vi "uService GUI.vi"(8 "error in (no error)":errorcluster, 11 "uService Template in":refnum<class "Common GUI v3.lvclass">) -> (3 "uService Template out":refnum<class "Common GUI v3.lvclass">)   [LabVIEW 2026, in "TALOS.lvlib" / "Common GUI v3.lvlib" / "Common GUI v3.lvclass"]
uses:
  Common GUI v3.lvclass
  C:/LabVIEW Code/TALOS/talos/Father of all uServices/Father of all uServices/Father of all uServices.lvclass
  Ancestor/Ancestor/Ancestor.lvclass/Ancestor.ctl
  Support VIs/Substitute Error.vi
  Support VIs/Generate Error.vi
  FGV/Error Memory/Get Error Description.vi
  Support VIs/Get PC name.vi
  Ancestor/Ancestor/Read ID.vi
  Support VIs/Get Class Name.vi
  FGV/Error Memory/Error Memory Core.vi
  <vilib>/AdvancedString/Delimited String to 1D String Array.vi
  <vilib>/AdvancedString/Delimited String to 1D String Array (string).vi
  Support VIs/Circus Root Path.vi
  FGV/Error Memory/Error Crt Lvl checker.vi
  FGV/Error Memory/Error Memory Core.vi/40c8088d-b597-4017-91af-faa98e00292e.vi
  FGV/Error Memory/Error Memory Core.vi/d4a3ab98-063c-4e44-b43d-fbdcfe6c2be2.vi
  Father of all uServices/Father of all uServices/Father of all uServices.lvclass
  C:/LabVIEW Code/TALOS/builds/Actor Framework PPL/Actor Framework.lvlibp/1abvi3w/vi.lib/ActorFramework/Actor/Actor.lvclass
  builds/Actor Framework PPL/Actor Framework.lvlibp/1abvi3w/vi.lib/ActorFramework/Actor/Read Self Enqueuer.vi
  builds/Actor Framework PPL/Actor Framework.lvlibp/1abvi3w/vi.lib/ActorFramework/Stop Msg/Send Normal Stop.vi
  Support VIs/Global Memory.vi
  <vilib>/Utility/LVClass/Get LV Class Name.vi
  Support VIs/Is in Packed Library.vi
  Support VIs/TALOS Root path.vi
  Support VIs/Read CSV worksheet.vi
  Support VIs/Global Constants.vi
  <vilib>/Utility/error.llb/General Error Handler.vi
  Support VIs/Error Log.vi
  Ancestor/Ancestor/Ancestor.lvclass
  <vilib>/Comparison/Equal/Equal Functor/Equal Functor.lvclass
panel:
  in  "Example":bool
  out "Safe Mode":bool
  in  "Stop":bool
  out "uService ID":string
  # "NOTHING!"
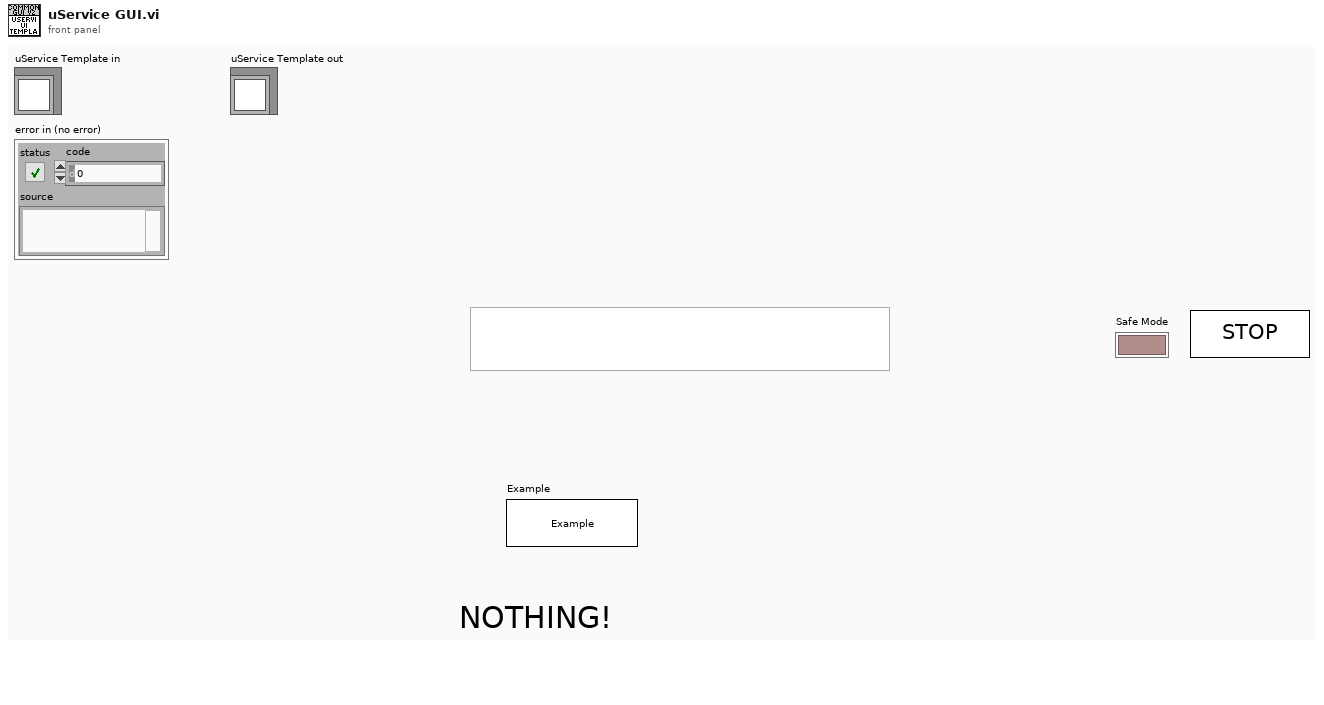
[diagram p1: front panel]
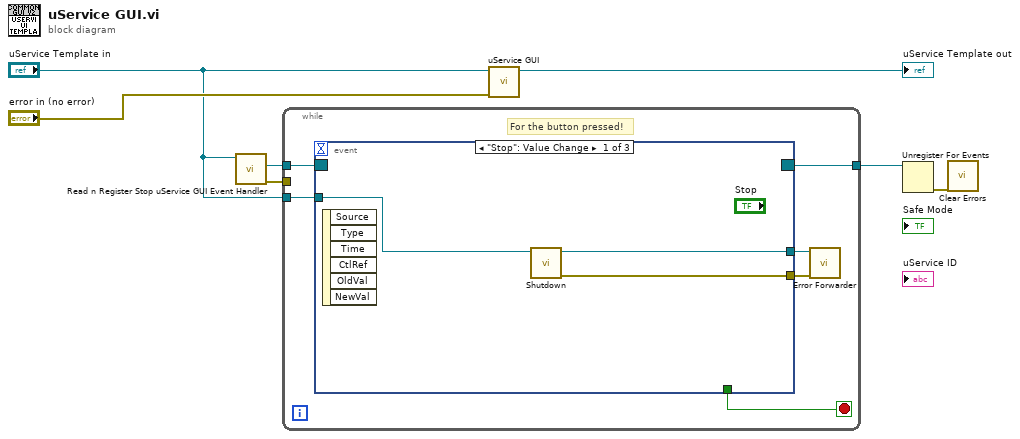
[diagram p0: block diagram]
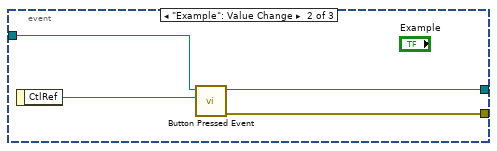
[diagram p2: hidden frame]
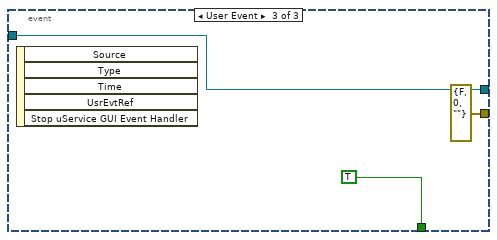
[diagram p3: hidden frame]
diagram:
  n1 = call-dynamic "Read n Register Stop uService GUI Event Handler .vi"("uService Template in"="uService Template in") -> ("error out"=w4:errorcluster, "Stop uService GUI Event Ref"=w3:refnum<event-registration>)  [unwired: 8 in, 1 out]
  n2 = while {
    tunnel: [w13] -> w5
    tunnel: w4 -> [_]
    tunnel: "uService Template in" -> [w11]
    tunnel: w3 -> [w10]
    stop <- w12 stop-if-true
    # "For the button pressed!"
    n3 = event shown="[0] \"Stop\": Value Change" {
      selector: w10 -> [_ _ _]
      dyn-events: [_ _ _] -> w13
      timeout: _ -> [_ _ _]
      tunnel: w11 -> [w16 w20 w22]
      tunnel: [_ _ TRUE] -> w12
      tunnel: [w15 w18 w22] -> w9
      tunnel: [w14 w17 errorcluster {"status"=FALSE, "code"=0, "source"=""} ("error out")] -> w8
      event "Stop": Value Change {
        n4 = event-data() -> ()  [unwired: 1 in, 6 out]
        n5 = call "Shutdown.vi"("Father of all uServices in"=w16) -> ("error out"=w14:errorcluster, "Father of all uServices out"=w15:refnum<class "Common GUI v3.lvclass">)  [unwired: 9 in]
      }
      event "Example": Value Change {
        n6 = event-data() -> ("CtlRef"=w19:refnum<vi>)  [unwired: 1 in]
        n7 = call-dynamic "Button Pressed Event.vi"("CtlRef"=w19, "uService Template in"=w20) -> ("error out"=w17:errorcluster, "uService Template out"=w18:refnum<class "Common GUI v3.lvclass">)  [unwired: 8 in]
      }
      event User Event {
        n8 = event-data() -> ()  [unwired: 1 in, 5 out]
      }
    }
    n9 = call "Error Forwarder.vi"("error in (no error)"=w8, "Father of all uServices in"=w9) -> ()  [unwired: 10 in]
  }
  n10 = call-parent "uService GUI.vi"("error in (no error)"="error in (no error)", "uService Template in"="uService Template in") -> ("uService Template out"=→"uService Template out":refnum<class "Common GUI v3.lvclass">)  [unwired: 9 in]
  n11 = Unregister For Events(event registration refnum=w5) -> (error out=w1:errorcluster)  [unwired: 1 in]
  n12 = call <vilib>:"Clear Errors.vi"("error in (no error)"=w1) -> ()  [unwired: 5 in, 2 out]
